vi "Flatten Readable.vi"(11 "Readable.lvclass":refnum<class "Readable.lvclass">) -> ()   [LabVIEW 2012, in "Readable.lvclass"]
uses:
  Readable.lvclass
  Global/File Locations.vi
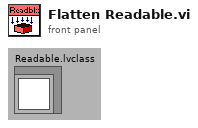
[diagram p1: front panel]
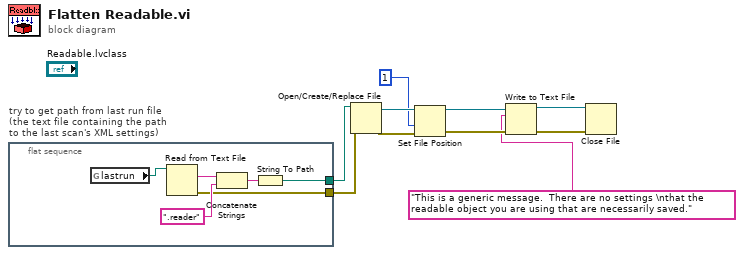
[diagram p0: block diagram]
diagram:
  n1 = flat-sequence "try to get path from last run file\n(the text file containing the path\nto the last scan's XML settings)" {
    tunnel: [w16] -> w5
    tunnel: [w11] -> w10
    frame #0 {
      n2 = global read "File Locations.vi" "lastrun"() -> (w15:path)
      n3 = Read from Text File(file (use dialog)=w15) -> (text=w14:string, error out=w11:errorcluster)  [unwired: 1 in, 4 out]
      n4 = Concatenate Strings(w14, ".reader") -> (w12:string)
      n5 = String To Path(string=w12) -> (path=w16:path)
    }
  }
  n6 = Open/Create/Replace File(file path (use dialog)=w5, error in=w10) -> (refnum out=w9:refnum<file>, error out=w7:errorcluster)  [unwired: 4 in, 1 out]
  n7 = Set File Position(refnum=w9, from (0:start)=1, error in=w7) -> (refnum out=w4:refnum<file>, error out=w6:errorcluster)  [unwired: 1 in]
  n8 = Write to Text File(file (use dialog)=w4, text="This is a generic message.  There are no settings \nthat the readable object you are using that are necessarily saved.", error in=w6) -> (refnum out=w3:refnum<file>, error out=w2:errorcluster)  [unwired: 1 in, 1 out]
  n9 = Close File(refnum=w3, error in=w2) -> ()  [unwired: 2 out]
